vi "daq.io Embedded Machine Example.vi"(8 "error in":errorcluster) -> (0 "error out":errorcluster)   [LabVIEW 2013, in "daqio minimal.lvlib"]
doc: "This interactive example demonstrates how an NI Embedded device can used for continuous monitoring with daq.io. Tags and Events in this example are written on user demand but could also be triggered by monitored values. \n\nTo get started, <b>drag this example onto a Real-Time target in the Project Explorer, enter your credentials in the block diagram</b> and run it interactively. You can also build an Executable and run it upon startup.\n\nClicking \"Create Dashboard\" will generate a dashboard for this device on daq.io.\n\nThe NI System Configuration API is being used to monitor the status of the Embedded device. Please make sure its libraries are installed on the Embedded Device to get the best experience."
uses:
  daqio minimal.lvlib
  _typedefs/update-button.ctl
  _typedefs/trigger-button.ctl
  _typedefs/dashboard-button.ctl
  _typedefs/daqio-Credentials.ctl
  _typedefs/exmpl-states.ctl
  _typedefs/connection_FGV_commands.ctl
  _typedefs/daqio-reconnect-status.ctl
  _typedefs/daqio-Buffer-Commands.ctl
  <vilib>/nisyscfg/Close (System).vi
  _subs/daqio_Write_Multiple_single_Timestamp.vi
  <resource>/objmgr/nisysapi.rc
  <vilib>/nisyscfg/nisyscfg.lvlib
panel:
  out "Setpoint":dbl(slide) scale=0.0..150.0
  out "shutdown":bool
  in  "Create Dashboard":T1
  out "Log":string[](array[string])
  in  "Stop":bool
  in  "Fire Event":T2
  in  "Select Event":u16(ring) items=["Safety Hood Status", "Manual Operation", "Shutting Down"]
  out "Time Stamp sent":timestamp
  in  "Event Data":string
  in  "Update Tags":T3
  out "connected":bool
  out "Speed (RPM)":dbl(knob) scale=0.0..2000.0
  out "Temperature Data":dbl(graph)
  out "RAM":dbl(slide) scale=0.0..100.0
  out "CPU":dbl(slide) scale=0.0..100.0
  in  "Value 3":string="1234-abc"
  in  "Value 2":string="XYZ 3000 Plus"
  in  "Tag 3":string="Serial Number"
  in  "Tag 2":string="Type"
  in  "Value 1":string="47.615459, -122.323804"
  in  "Tag 1":string="Location"
  out "Device Key":string
  out "Device Type Key":string
  out "Dashboard URL - copy and open in your web browser":string
  # "Get your free account at daq.io first: sign up at daq.io."
  # "This Machine"
  # "(autogenerated in this example)"
  # "Please enter your \ncredentials in the \nblock diagram."
  # "Device Tags"
  # "Use device tags to describe \nspecific parameters for each\ndevice. These can include the \nlocation, the serial number or\nother machine or location-\nspecific information. These\nfields are fully user-defined."
  # "Device Events"
  # "Use device events to signal\nany local event to daq.io. These\ncould include mechanical events\n(e.g. \"safety latch released\") or \nany change on the device that\nneeds to be tracked."
  # "Device Live Data Channels"
  # "Use device channels to transfer\ntime series data. All channels \nof the device will be visible in \nthe online data viewer. You \ncan build your own dashboard \nin the webbrowser and link it\nto exisiting channels. Clicking\n\"Create Dashboard\" will\ngenerate a dashboard \nfor this example."
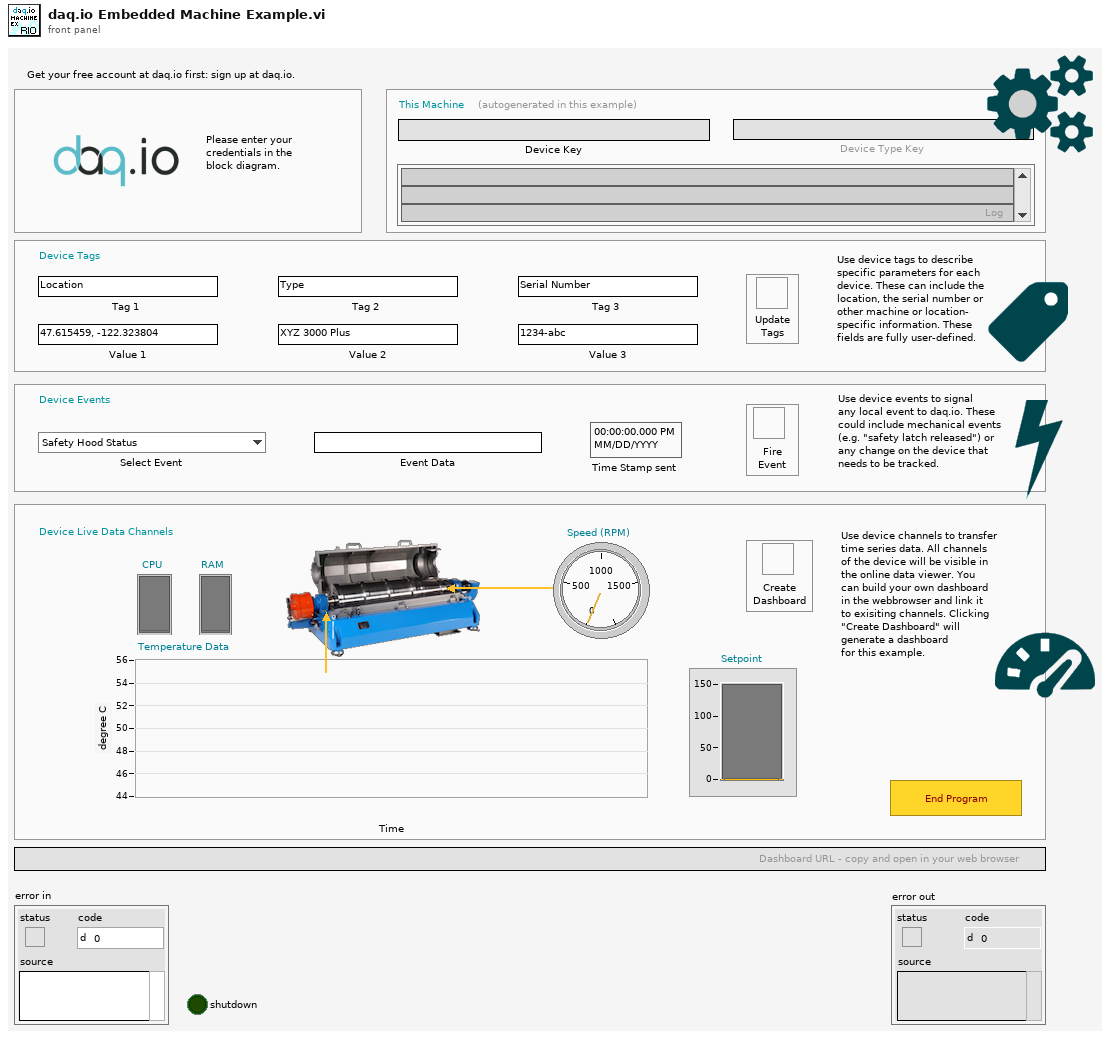
[diagram p1: front panel]
types:
  T1 = typedef "daqio minimal.lvlib/dashboard-button.ctl" = bool
  T2 = typedef "daqio minimal.lvlib/trigger-button.ctl" = bool
  T3 = typedef "daqio minimal.lvlib/update-button.ctl" = bool
  T4 = typedef "daqio minimal.lvlib/exmpl-states.ctl" = enum16{"idle", "time series", "fire events", "update tags", "end program", "create waveform", "create dashboard"}
  T5 = typedef "daqio minimal.lvlib/daqio-Credentials.ctl" = cluster{"User Name (email)":string, "Password":string}
  T6 = typedef "daqio minimal.lvlib/daqio-Type.ctl" = cluster{"daq.io ref":T7, "daq.io API Base":string, "Device Type Key":string, "Device Key":string, "Account ID":string, "online":bool, "SSL":bool}
  T7 = typedef "LabVIEWHTTPClient.lvlib/ClientHandle.ctl" = refnum<k1>
  T8 = typedef "daqio minimal.lvlib/connection_FGV_commands.ctl" = enum16{"Set Conn Stat", "Save Type", "Get Type from File", "Set Type", "Set Buffer", "Get"}
  T9 = typedef "daqio minimal.lvlib/daqio-reconnect-status.ctl" = enum16{"Reconnect success", "Reconnect failed", "Connected", "Offline"}
  T10 = typedef "daqio minimal.lvlib/daqio-Buffer-Commands.ctl" = enum16{"Add to Buffer", "Post from Buffer", "Clear Buffer", "Init"}
  T11 = enum8{"Enabled", "Disabled", "Disabled and Grayed Out"}
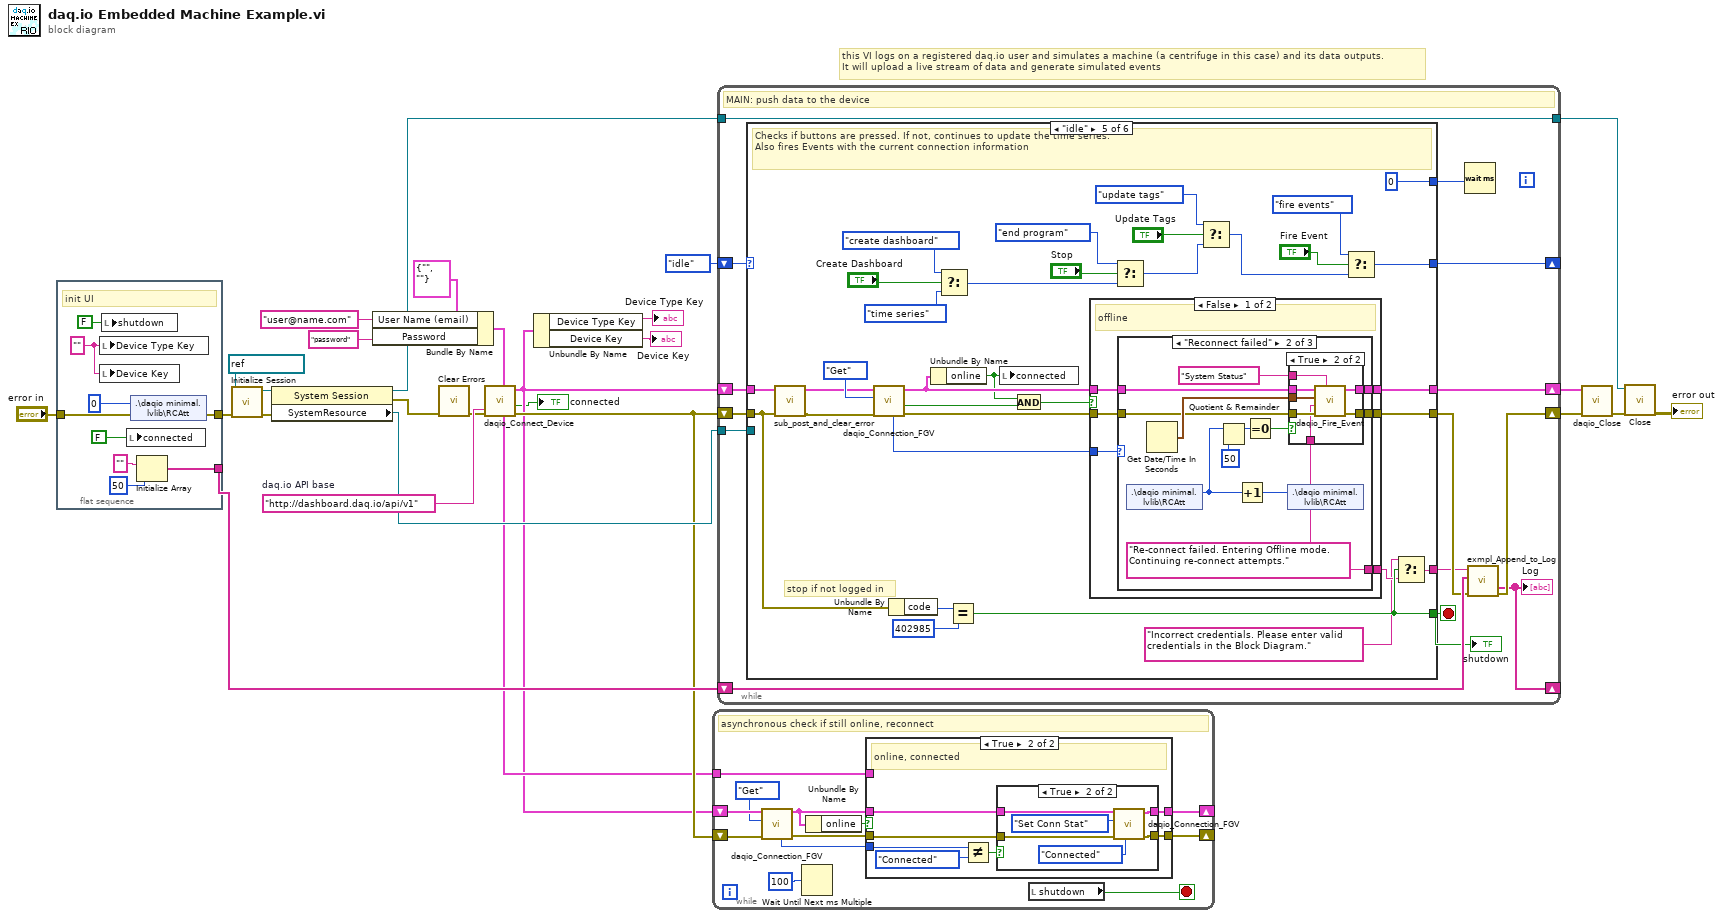
[diagram p0: block diagram]
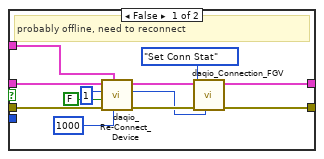
[diagram p2: hidden frame]
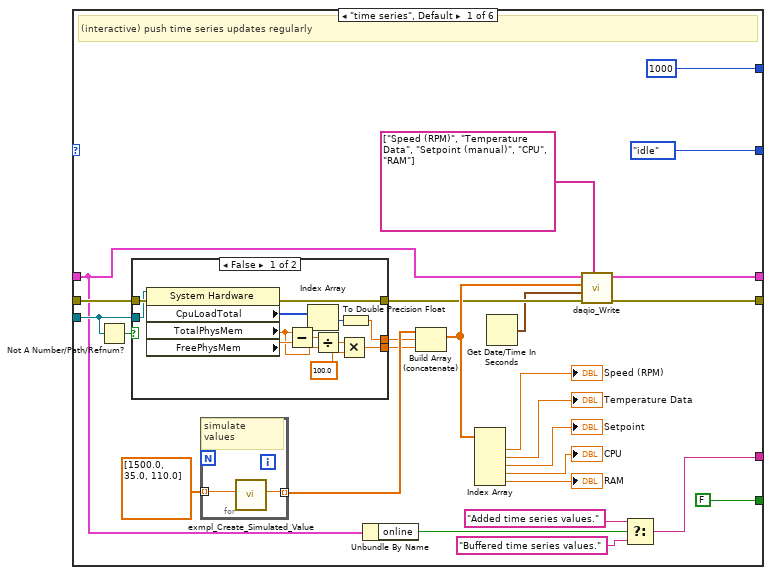
[diagram p4: hidden frame]
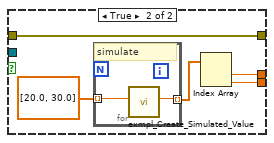
[diagram p5: hidden frame]
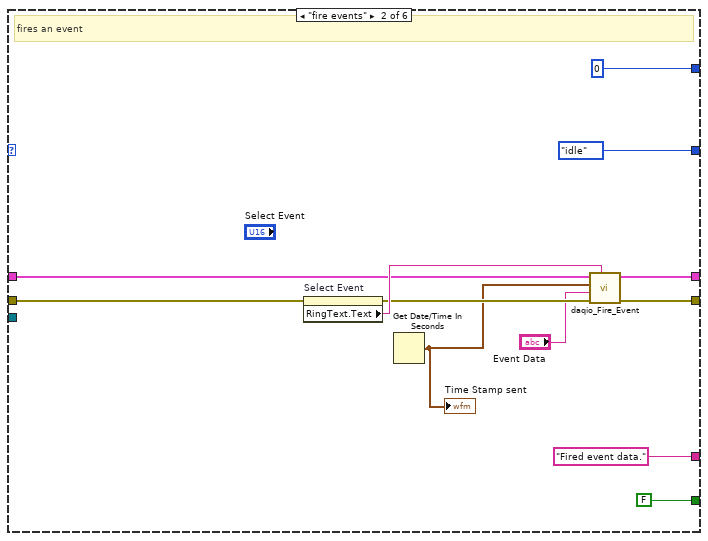
[diagram p6: hidden frame]
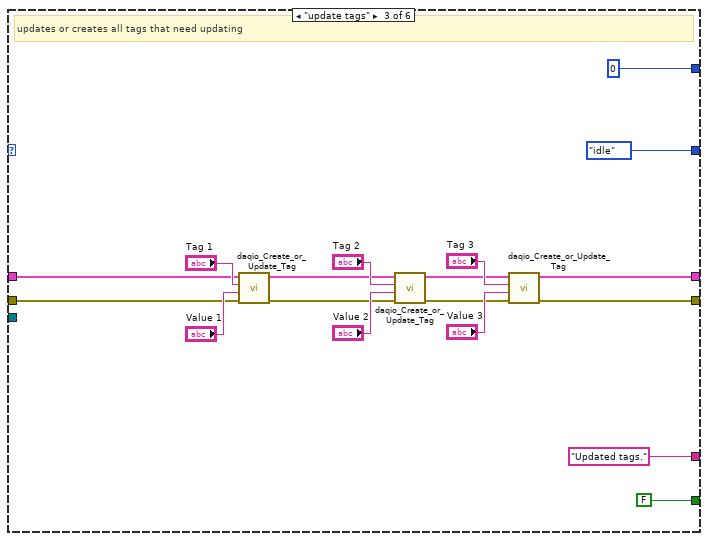
[diagram p7: hidden frame]
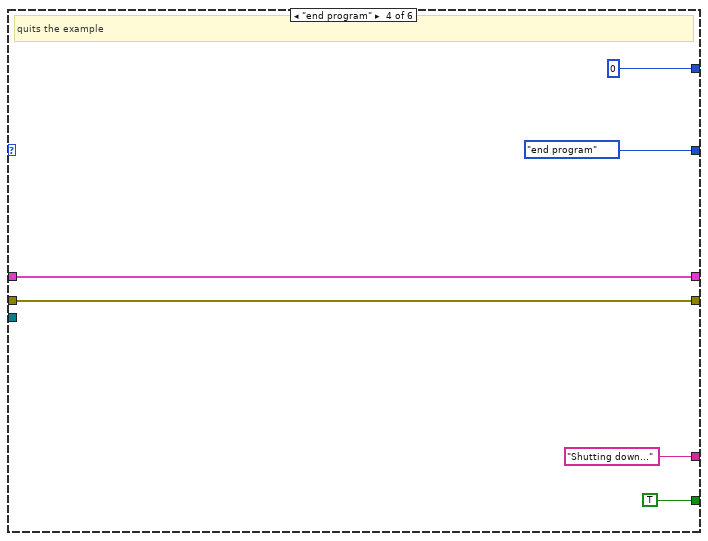
[diagram p8: hidden frame]
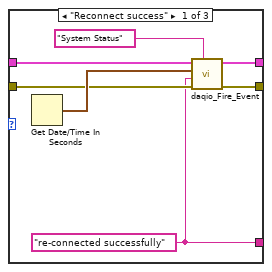
[diagram p9: hidden frame]
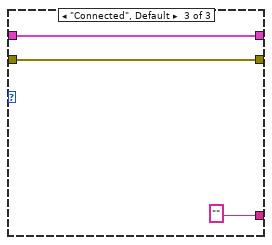
[diagram p11: hidden frame]
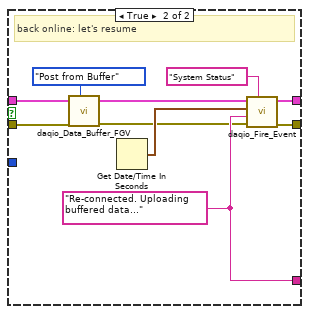
[diagram p12: hidden frame]
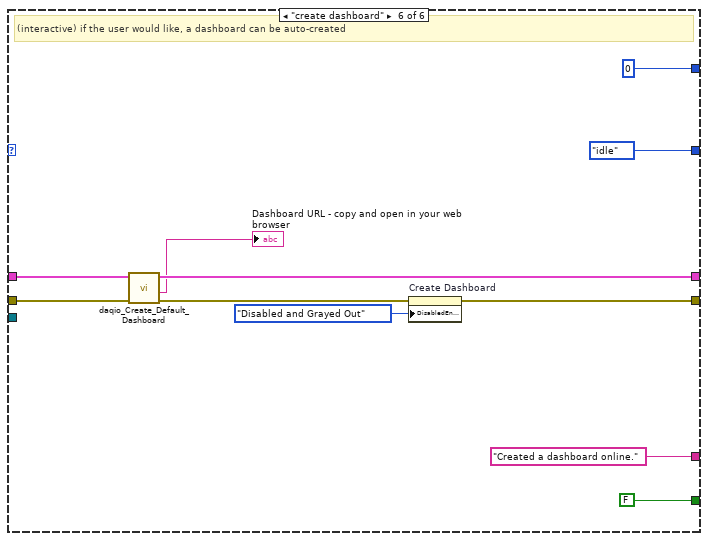
[diagram p13: hidden frame]
diagram:
  w22 = "http://dashboard.daq.io/api/v1"  # daq.io API base
  # "this VI logs on a registered daq.io user and simulates a machine (a centrifuge in this case) and its data outputs. \nIt will upload a live stream of data and generate simulated events"
  n1 = flat-sequence {
    tunnel: [w28] -> w19
    tunnel: "error in" -> [w30]
    tunnel: [w31] -> w6
    frame #0 {
      w35 = "" ("log")
      # "init UI"
      n2 = local write "Device Type Key"(w35) -> ()
      n3 = local write "Device Key"(w35) -> ()
      n4 = local write "shutdown"(FALSE ("shutdown")) -> ()
      n5 = local write "connected"(FALSE ("connected to daq.io")) -> ()
      n6 = shared-variable ".\\daqio minimal.lvlib\\RCAtt"(0 ("RCAtt"), error in=w30) -> (error out=w28:errorcluster)
      n7 = Initialize Array("" ("log"), 50 ("dimension size")) -> (w31:string[])
    }
  }
  n8 = call <vilib>:"Initialize Session.vi"("error in (no error)"=w19, "target (localhost)"=refnum<k21> "localhost" ("Embedded Target (self)")) -> ("error out"=w13:errorcluster, "session out"=w11:refnum<k21>)  [unwired: 8 in]
  n9 = property class="System Session"(reference=w11, error in=w13) -> (reference out=w10:refnum<k21>, error out=w12:errorcluster, "SystemResource"=w14:refnum<k20>)
  n10 = Bundle By Name(cluster=T5 {"User Name (email)"="", "Password"=""} ("daq.io Credentials"), "User Name (email)"="user@name.com" ("User Name"), "Password"="password") -> (w4:T5)
  n11 = call <vilib>:"Clear Errors.vi"("error in (no error)"=w12) -> ("error out"=w2:errorcluster)  [unwired: 6 in]
  n12 = call "daqio_Connect_Device.vi"("daq.io API base"=w22, "error in (no error)"=w2, "Credentials"=w4) -> ("error out"=w5:errorcluster, "connected successfully?"=→"connected":bool, "daq.io type out"=w3:T6)  [unwired: 5 in, 1 out]
  n13 = Unbundle By Name(w3) -> ("Device Type Key"=→"Device Type Key":string, "Device Key"=→"Device Key":string)
  n14 = while {
    tunnel: w4 -> [w45]
    shift-right: [w39] -> _
    shift-left: w5 -> [w43]
    shift-right: [w40] -> _
    shift-left: w3 -> [w44]
    stop <- w47 stop-if-true
    # "asynchronous check if still online, reconnect"
    n15 = call "daqio_Connection_FGV.vi"("error in"=w43, "Enum"=connection_FGV_commands."Get", "daq.io type in"=w44) -> ("error out"=w41:errorcluster, "daq.io type out"=w37:T6, "Connection Status out"=w36:T9)  [unwired: 5 in, 1 out]
    n16 = Wait Until Next ms Multiple(millisecond multiple=u32 100) -> ()  [unwired: 1 out]
    n17 = Unbundle By Name(w37) -> ("online"=w38:bool)
    n18 = case shown="True" w38 {
      tunnel: w45 -> [w59 _]
      tunnel: w41 -> [w56 w61]
      tunnel: [w51 w64] -> w40
      tunnel: [w50 w63] -> w39
      tunnel: w37 -> [w49 w62]
      tunnel: w36 -> [_ w66]
      frame False {
        # "probably offline, need to reconnect"
        n19 = call "daqio_Re-Connect_Device.vi"("re-connect timeouts"=u32 1000, "Credentials"=w59, "error in"=w56, "override any errors"=FALSE, "re-connect attempts"=1, "daq.io type in"=w49) -> ("error out"=w55:errorcluster, "status"=w52:T9, "daq.io type out"=w54:T6)  [unwired: 3 in]
        n20 = call "daqio_Connection_FGV.vi"("Connection Status in"=w52, "error in"=w55, "Enum"=connection_FGV_commands."Set Conn Stat", "daq.io type in"=w54) -> ("error out"=w50:errorcluster, "daq.io type out"=w51:T6)  [unwired: 4 in, 2 out]
      }
      frame True {
        # "online, connected"
        n21 = Not Equal?(x=w66, y=daqio-reconnect-status."Connected") -> (x != y?=w60:bool)
        n22 = case shown="True" w60 {
          tunnel: [w68 w74] -> w64
          tunnel: [w67 w73] -> w63
          tunnel: w62 -> [w68 w72]
          tunnel: w61 -> [w67 w71]
          frame False {
          }
          frame True {
            n23 = call "daqio_Connection_FGV.vi"("Connection Status in"=daqio-reconnect-status."Connected", "error in"=w71, "Enum"=connection_FGV_commands."Set Conn Stat", "daq.io type in"=w72) -> ("error out"=w73:errorcluster, "daq.io type out"=w74:T6)  [unwired: 4 in, 2 out]
          }
        }
      }
    }
    n24 = local read "shutdown"() -> (w47:bool)
  }
  n25 = while {
    shift-right: [w80] -> w26
    shift-left: w5 -> [w77]
    shift-right: [w88] -> w24
    shift-left: w3 -> [w78]
    shift-right: [w86] -> _
    shift-left: exmpl-states."idle" -> [w87]
    tunnel: w14 -> [w84]
    tunnel: [w83] -> w16
    tunnel: w10 -> [w83]
    shift-right: [w79] -> _
    shift-left: w6 -> [w82]
    stop <- w75 stop-if-true
    # "MAIN: push data to the device"
    n26 = case shown="\"idle\"" w87 {
      tunnel: w78 -> [w89 w144 w155 w169 w179 w258]
      tunnel: w77 -> [w107 w143 w154 w168 w178 w257]
      tunnel: [w92 w141 w152 w169 w188 w256] -> w88
      tunnel: [w91 w142 w153 w168 w187 w252] -> w81
      tunnel: [exmpl-states."idle" exmpl-states."idle" exmpl-states."idle" exmpl-states."end program" w201 exmpl-states."idle"] -> w86
      tunnel: [FALSE FALSE FALSE TRUE w175 FALSE] -> w75
      tunnel: [u32 1000 ("milliseconds to wait") u32 0 ("milliseconds to wait") u32 0 ("milliseconds to wait") u32 0 ("milliseconds to wait") u32 0 ("milliseconds to wait") u32 0 ("milliseconds to wait")] -> w85
      tunnel: [w99 "Fired event data." ("log") "Updated tags." ("log") "Shutting down..." ("log") w173 "Created a dashboard online." ("log")] -> w76
      tunnel: w84 -> [w105 _ _ _ _ _]
      frame "time series", Default {
        # "(interactive) push time series updates regularly"
        n27 = Not A Number/Path/Refnum?(number/path/refnum=w105) -> (NaN/Path/Refnum?=w104:bool)
        n28 = case shown="False" w104 {
          tunnel: w107 -> [w126 w127]
          tunnel: w105 -> [w125 _]
          tunnel: [w124 w127] -> w94
          tunnel: [w120 w128] -> w106
          tunnel: [w118 w129] -> w103
          frame False {
            n29 = property class="System Hardware"(reference=w125, error in=w126) -> (error out=w124:errorcluster, "CpuLoadTotal"=w123:u32[], "TotalPhysMem"=w115:dbl, "FreePhysMem"=w116:dbl)  [unwired: 1 out]
            n30 = Subtract(x=w115, y=w116) -> (x-y=w117:dbl)
            n31 = Index Array(array=w123) -> (element=w119:u32)  [unwired: 1 in]
            n32 = Divide(x=w117, y=w115) -> (x/y=w122:dbl)
            n33 = Multiply(x=w122, y=100.0) -> (x*y=w120:dbl)
            n34 = To Double Precision Float(number=w119) -> (double precision float=w118:dbl)
          }
          frame True {
            n35 = for {
              tunnel: [w133] -> w130 mode=indexing
              tunnel: dbl[] [20.0, 30.0] -> [w132] mode=indexing
              # "simulate"
              n36 = call "exmpl_Create_Simulated_Value.vi"("offset"=w132) -> ("Numeric"=w133:dbl)  [unwired: 9 in, 1 out]
            }
            n37 = Index Array(array=w130) -> (element #1=w129:dbl, element #2=w128:dbl)  [unwired: 2 in]
          }
        }
        n38 = for {
          tunnel: [w135] -> w114 mode=indexing
          tunnel: dbl[] [1500.0, 35.0, 110.0] -> [w134] mode=indexing
          # "simulate\nvalues"
          n39 = call "exmpl_Create_Simulated_Value.vi"("offset"=w134) -> ("Numeric"=w135:dbl)  [unwired: 9 in, 1 out]
        }
        n40 = Unbundle By Name(w89) -> ("online"=w102:bool)
        n41 = Build Array (concatenate)(w114, w103, w106) -> (w95:dbl[])
        n42 = Index Array(array=w95) -> (element #1=→"Speed (RPM)":dbl, element #2=→"Temperature Data":dbl, element #3=→"Setpoint":dbl, element #4=→"CPU":dbl, element #5=→"RAM":dbl)  [unwired: 5 in]
        n43 = Get Date/Time In Seconds() -> (seconds since 1Jan1904=w90:timestamp)
        n44 = call-poly "daqio_Write.vi"("daq.io Device Channel Keys"=string[] ["Speed (RPM)", "Temperature Data", "Setpoint (manual)", "CPU", "RAM"], "error in (no error)"=w94, "Timestamp"=w90, "Values"=w95, "daq.io type in"=w89) -> ("error out"=w91:errorcluster, "daq.io type out"=w92:T6)  [unwired: 5 in]
        n45 = Select(t="Added time series values." ("log"), s=w102, f="Buffered time series values." ("log")) -> (s? t:f=w99:string)
      }
      frame "fire events" {
        # "fires an event"
        n46 = property on="Select Event" class="Ring (strict)"(error in=w143) -> (error out=w146:errorcluster, "RingText.Text"=w147:string)  [unwired: 1 in, 1 out]
        n47 = Get Date/Time In Seconds() -> (seconds since 1Jan1904=w136:timestamp)
        "Time Stamp sent" <- w136
        n48 = call "daqio_Fire_Event.vi"("Event Key"=w147, "error in (no error)"=w146, "Event Value"="Event Data", "Event Date and Time"=w136, "daq.io type in"=w144) -> ("error out"=w142:errorcluster, "daq.io type out"=w141:T6)  [unwired: 5 in]
      }
      frame "update tags" {
        # "updates or creates all tags that need updating"
        n49 = call "daqio_Create_or_Update_Tag.vi"("error in (no error)"=w154, "Tag Value"="Value 1", "Tag Key"="Tag 1", "daq.io type in"=w155) -> ("error out"=w159:errorcluster, "daq.io type out"=w156:T6)  [unwired: 5 in, 1 out]
        n50 = call "daqio_Create_or_Update_Tag.vi"("error in (no error)"=w159, "Tag Value"="Value 2", "Tag Key"="Tag 2", "daq.io type in"=w156) -> ("error out"=w158:errorcluster, "daq.io type out"=w157:T6)  [unwired: 5 in, 1 out]
        n51 = call "daqio_Create_or_Update_Tag.vi"("error in (no error)"=w158, "Tag Value"="Value 3", "Tag Key"="Tag 3", "daq.io type in"=w157) -> ("error out"=w153:errorcluster, "daq.io type out"=w152:T6)  [unwired: 5 in, 1 out]
      }
      frame "end program" {
        # "quits the example"
      }
      frame "idle" {
        # "stop if not logged in"
        # "Checks if buttons are pressed. If not, continues to update the time series. \nAlso fires Events with the current connection information"
        n52 = call "sub_post_and_clear_error.vi"("error in (no error)"=w178, "daq.io type in"=w179) -> ("error out"=w181:errorcluster, "daq.io type out"=w180:T6)  [unwired: 8 in]
        n53 = call "daqio_Connection_FGV.vi"("error in"=w181, "Enum"=connection_FGV_commands."Get", "daq.io type in"=w180) -> ("error out"=w189:errorcluster, "Buffered Data exists?"=w185:bool, "daq.io type out"=w184:T6, "Connection Status out"=w182:T9)  [unwired: 5 in]
        n54 = Unbundle By Name(w178) -> ("code"=w177:i32)
        n55 = Unbundle By Name(w184) -> ("online"=w183:bool)
        n56 = Select(t=exmpl-states."create dashboard", s="Create Dashboard", f=exmpl-states."time series") -> (s? t:f=w191:T4)
        n57 = Equal?(x=w177, y=402985) -> (x = y?=w175:bool)
        n58 = local write "connected"(w183) -> ()
        n59 = And(x=w183, y=w185) -> (x .and. y?=w186:bool)
        n60 = case shown="False" w186 {
          tunnel: w184 -> [w206 w250]
          tunnel: w189 -> [w207 w249]
          tunnel: [w210 w247] -> w174
          tunnel: [w209 w243] -> w188
          tunnel: [w208 w242] -> w187
          tunnel: w182 -> [w205 _]
          frame False {
            # "offline"
            n61 = case shown="\"Reconnect failed\"" w205 {
              tunnel: [w211 w223 ""] -> w210
              tunnel: [w215 w224 w240] -> w209
              tunnel: [w214 w225 w239] -> w208
              tunnel: w207 -> [w213 w227 w239]
              tunnel: w206 -> [w212 w226 w240]
              frame "Reconnect success" {
                w211 = "re-connected successfully"
                n62 = Get Date/Time In Seconds() -> (seconds since 1Jan1904=w217:timestamp)
                n63 = call "daqio_Fire_Event.vi"("Event Key"="System Status", "error in (no error)"=w213, "Event Value"=w211, "Event Date and Time"=w217, "daq.io type in"=w212) -> ("error out"=w214:errorcluster, "daq.io type out"=w215:T6)  [unwired: 5 in]
              }
              frame "Reconnect failed" {
                w223 = "Re-connect failed. Entering Offline mode. Continuing re-connect attempts."
                n64 = shared-variable ".\\daqio minimal.lvlib\\RCAtt"() -> (w219:i32)  [unwired: 1 in, 1 out]
                n65 = Get Date/Time In Seconds() -> (seconds since 1Jan1904=w229:timestamp)
                n66 = Quotient & Remainder(x=w219, y=50) -> (x-y*floor(x/y)=w222:i32)  [unwired: 1 out]
                n67 = Increment(x=w219) -> (x+1=w218:i32)
                n68 = Equal To 0?(x=w222) -> (x = 0?=w221:bool)
                n69 = shared-variable ".\\daqio minimal.lvlib\\RCAtt"(w218) -> ()  [unwired: 1 in, 1 out]
                n70 = case shown="True" w221 {
                  tunnel: w229 -> [_ w238]
                  tunnel: "System Status" ("Event Key") -> [_ w237]
                  tunnel: w227 -> [w230 w236]
                  tunnel: w226 -> [w231 w235]
                  tunnel: [w230 w234] -> w225
                  tunnel: [w231 w233] -> w224
                  tunnel: w223 -> [_ w232]
                  frame False {
                  }
                  frame True {
                    n71 = call "daqio_Fire_Event.vi"("Event Key"=w237, "error in (no error)"=w236, "Event Value"=w232, "Event Date and Time"=w238, "daq.io type in"=w235) -> ("error out"=w234:errorcluster, "daq.io type out"=w233:T6)  [unwired: 5 in]
                  }
                }
              }
              frame "Connected", Default {
              }
            }
          }
          frame True {
            w247 = "Re-connected. Uploading buffered data..."
            # "back online: let's resume"
            n72 = call "daqio_Data_Buffer_FGV.vi"("Buffer Command"=daqio-Buffer-Commands."Post from Buffer", "error in (no error)"=w249, "daq.io type in"=w250) -> ("error out"=w245:errorcluster, "daq.io type out"=w246:T6)  [unwired: 7 in]
            n73 = Get Date/Time In Seconds() -> (seconds since 1Jan1904=w248:timestamp)
            n74 = call "daqio_Fire_Event.vi"("Event Key"="System Status", "error in (no error)"=w245, "Event Value"=w247, "Event Date and Time"=w248, "daq.io type in"=w246) -> ("error out"=w242:errorcluster, "daq.io type out"=w243:T6)  [unwired: 5 in]
          }
        }
        n75 = Select(t=exmpl-states."end program", s="Stop", f=w191) -> (s? t:f=w196:T4)
        n76 = Select(t=exmpl-states."update tags", s="Update Tags", f=w196) -> (s? t:f=w202:T4)
        n77 = Select(t=exmpl-states."fire events", s="Fire Event", f=w202) -> (s? t:f=w201:T4)
        n78 = Select(t="Incorrect credentials. Please enter valid credentials in the Block Diagram.", s=w175, f=w174) -> (s? t:f=w173:string)
      }
      frame "create dashboard" {
        # "(interactive) if the user would like, a dashboard can be auto-created"
        n79 = call "daqio_Create_Default_Dashboard.vi"("error in (no error)"=w257, "daq.io type in"=w258) -> ("error out"=w253:errorcluster, "Dashboard URL"=→"Dashboard URL - copy and open in your web browser":string, "daq.io type out"=w256:T6)  [unwired: 6 in, 1 out]
        n80 = property on="Create Dashboard" class="Bool"(error in=w253, "DisabledEnum"=T11."Disabled and Grayed Out" ("Disabled")) -> (error out=w252:errorcluster)  [unwired: 1 in, 1 out]
      }
    }
    "shutdown" <- w75
    n81 = Wait (ms)(milliseconds to wait=w85) -> ()  [unwired: 1 out]
    n82 = call "exmpl_Append_to_Log.vi"("error in (no error)"=w81, "Log Array in"=w82, "Log Message"=w76) -> ("error out"=w80:errorcluster, "Log Array out"=w79:string[])  [unwired: 7 in]
    "Log" <- w79
  }
  n83 = call "daqio_Close.vi"("error in (no error)"=w26, "daq.io type"=w24) -> ("error out"=w18:errorcluster)  [unwired: 9 in]
  n84 = call-poly <vilib>:"Close.vi"("error in (no error)"=w18, "session in"=w16) -> ("error out"=→"error out":errorcluster)  [unwired: 9 in]
